vi "Arithmetics.vi"(0 "Operation.lvclass":refnum<class "Operation.lvclass">, 1 "Numeric 1":dbl, 4 "Numeric 2":dbl, 5 "multiplier":dbl) -> (14 "result":dbl)   [LabVIEW 2024]
uses:
  Operation.lvclass
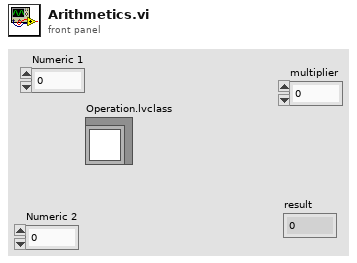
[diagram p1: front panel]
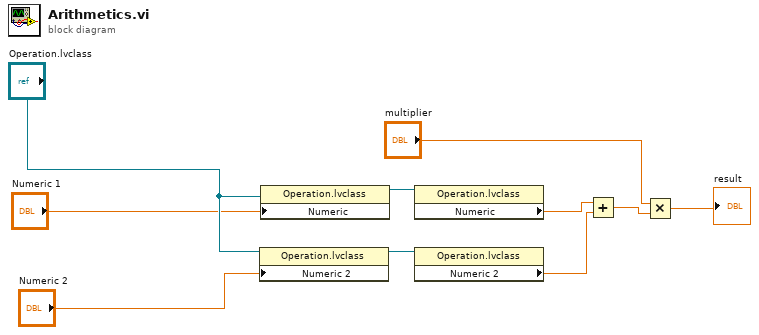
[diagram p0: block diagram]
diagram:
  n1 = property class="Operation.lvclass"(reference="Operation.lvclass", "Numeric 2"="Numeric 2") -> (reference out=w7:refnum<class "Operation.lvclass">)  [unwired: 1 in, 1 out]
  n2 = property class="Operation.lvclass"(reference="Operation.lvclass", "Numeric"="Numeric 1") -> (reference out=w6:refnum<class "Operation.lvclass">)  [unwired: 1 in, 1 out]
  n3 = property class="Operation.lvclass"(reference=w6) -> ("Numeric"=w5:dbl)  [unwired: 1 in, 2 out]
  n4 = property class="Operation.lvclass"(reference=w7) -> ("Numeric 2"=w4:dbl)  [unwired: 1 in, 2 out]
  n5 = Add(x=w5, y=w4) -> (x+y=w3:dbl)
  n6 = Multiply(x="multiplier", y=w3) -> (x*y=→"result":dbl)
